vi "DAQ Activate Output.vi"(5 "error in":errorcluster, 6 "lines":tag, 7 "data":bool) -> (1 "error out":errorcluster, 3 "task out":refnum<k21>)   [LabVIEW 2022 SP3]
uses:
  <vilib>/DAQmx/write.llb/DAQmx Write (Digital Bool 1Line 1Point).vi
  <vilib>/DAQmx/miscellaneous.llb/DAQmx Fill In Error Info.vi
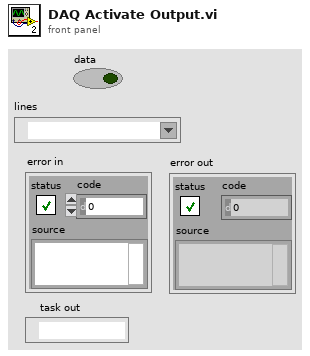
[diagram p1: front panel]
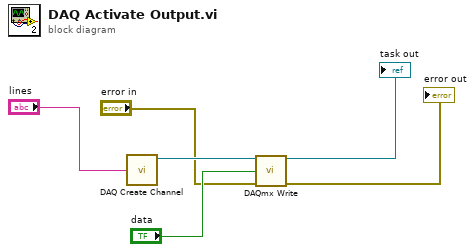
[diagram p0: block diagram]
diagram:
  n1 = call "DAQ Create Channel.vi"("lines"="lines") -> ("task out"=w6:refnum<k21>)  [unwired: 3 in, 1 out]
  n2 = call-poly <vilib>:"DAQmx Write.vi"("task/channels in"=w6, "data"="data", "error in"="error in") -> ("task out"=→"task out":refnum<k21>, "error out"=→"error out":errorcluster)  [unwired: 10 in, 1 out]
